vi "Golden Section 1D.vi"(4 "accuracy":dbl=1e-08 format="%.0e", 5 "formula":string="0", 6 "c (start)":dbl format="%.2f", 7 "b (start)":dbl format="%.2f", 8 "a (start)":dbl format="%.2f") -> (0 "error":i32, 1 "ticks":u32, 2 "f(minimum)":dbl format="%.2f", 3 "minimum":dbl format="%.2f")   [LabVIEW 2020, in "NI_Gmath.lvlib"]
doc: "Determines a local minimum of a given 1D function with the help of a bracketing of the minimum. The Golden Section Search method is used."
uses:
  <vilib>/gmath/NI_Gmath.lvlib
panel:
  # "Example:\n\n accuracy: 1E-8 \n a (start): 0.0 \n b (start): 0.5\n c (start): 1.0 \n formula: (x-(3/10))^2+1"
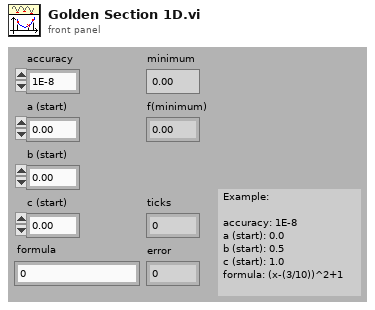
[diagram p1: front panel]
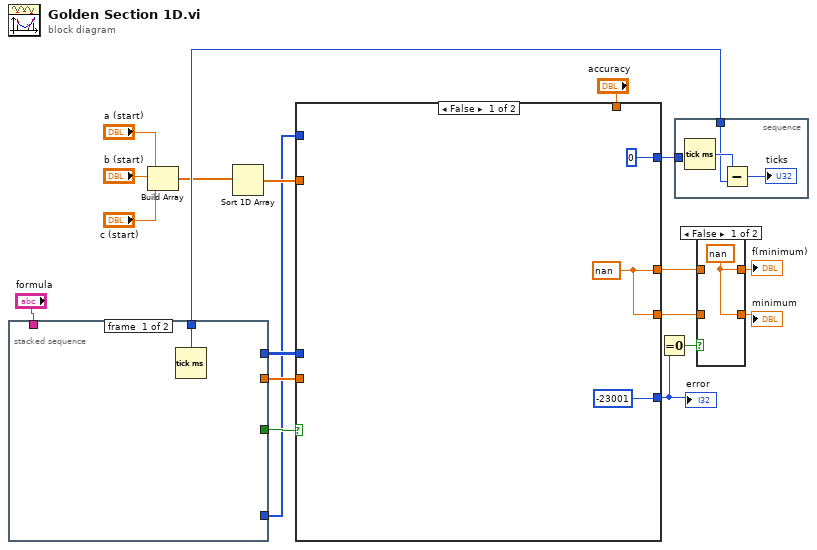
[diagram p0: block diagram]
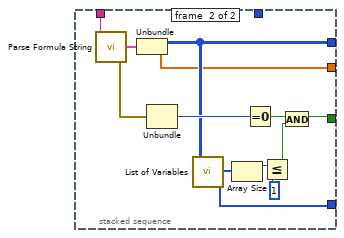
[diagram p3: hidden frame]
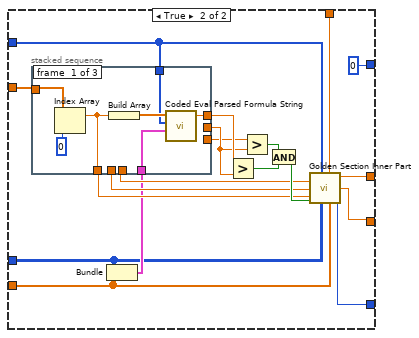
[diagram p4: hidden frame]
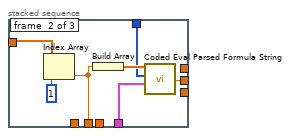
[diagram p5: hidden frame]
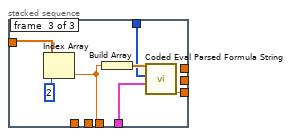
[diagram p6: hidden frame]
diagram:
  n1 = stacked-sequence {
    tunnel: [_ w32] -> w19
    tunnel: [w20 _] -> w18
    tunnel: "formula" -> [_ w26]
    tunnel: [_ w22] -> w3
    tunnel: [_ w21] -> w2
    tunnel: [_ w27] -> w1
    frame #0 {
      n2 = Tick Count (ms)() -> (millisecond timer value=w20:u32)
    }
    frame #1 {
      n3 = call <vilib>:"Parse Formula String.vi"("formula"=w26) -> ("error out"=w25:errorcluster, "Parsed Formula"=w23:cluster{"Table":i32[][], "Y Values":dbl[]})  [unwired: 1 in]
      n4 = Unbundle(w23) -> ("Table"=w22:i32[][], "Y Values"=w21:dbl[])
      n5 = Unbundle(w25) -> ("code"=w24:i32)  [unwired: 2 out]
      n6 = call <vilib>:"List of Variables.vi"("Table"=w22) -> ("List of variables"=w27:i32[])
      n7 = Array Size(array=w27) -> (size(s)=w28:i32)
      n8 = Equal To 0?(x=w24) -> (x = 0?=w31:bool)
      n9 = Less Or Equal?(x=w28, y=1) -> (x <= y?=w30:bool)
      n10 = And(x=w31, y=w30) -> (x .and. y?=w32:bool)
    }
  }
  n11 = Build Array("a (start)", "b (start)", "c (start)") -> (w14:dbl[])
  n12 = Sort 1D Array(array=w14) -> (sorted array=w13:dbl[])
  n13 = case shown="False" w19 {
    tunnel: w13 -> [_ w54]
    tunnel: [0 0] -> w12
    tunnel: [w34 w43] -> w8
    tunnel: [w34 w42] -> w6
    tunnel: [-23001 w41] -> w10
    tunnel: "accuracy" -> [_ w39]
    tunnel: w3 -> [_ w38]
    tunnel: w2 -> [_ w37]
    tunnel: w1 -> [_ w36]
    frame False {
      w34 = nan
      (unwired) 0
    }
    frame True {
      (unwired) 0
      n14 = Bundle("Table"=w38, "Y Values"=w37) -> (w40:cluster{"Table":i32[][], "Y Values":dbl[]})  [unwired: 1 in]
      n15 = stacked-sequence {
        tunnel: w54 -> [w61 w68 w75]
        tunnel: w36 -> [w56 w62 w70]
        tunnel: [w59 _ _] -> w53
        tunnel: [_ w66 _] -> w52
        tunnel: [_ _ w73] -> w51
        tunnel: [w58 _ _] -> w47
        tunnel: [_ w65 _] -> w46
        tunnel: [_ _ w72] -> w45
        tunnel: w40 -> [w55 w63 w69]
        frame #0 {
          n16 = Index Array(array=w61, index=0) -> (element=w58:dbl)
          n17 = Build Array(w58) -> (w57:dbl[])
          n18 = call <vilib>:"Coded Eval Parsed Formula String.vi"("Parsed Formula"=w55, "Variables"=w56, "X Values"=w57) -> ("y value"=w59:dbl)  [unwired: 1 in, 1 out]
        }
        frame #1 {
          n19 = Index Array(array=w68, index=1) -> (element=w65:dbl)
          n20 = Build Array(w65) -> (w64:dbl[])
          n21 = call <vilib>:"Coded Eval Parsed Formula String.vi"("Parsed Formula"=w63, "Variables"=w62, "X Values"=w64) -> ("y value"=w66:dbl)  [unwired: 1 in, 1 out]
        }
        frame #2 {
          n22 = Index Array(array=w75, index=2) -> (element=w72:dbl)
          n23 = Build Array(w72) -> (w71:dbl[])
          n24 = call <vilib>:"Coded Eval Parsed Formula String.vi"("Parsed Formula"=w69, "Variables"=w70, "X Values"=w71) -> ("y value"=w73:dbl)  [unwired: 1 in, 1 out]
        }
      }
      n25 = Greater?(x=w53, y=w52) -> (0:w50:bool)
      n26 = Greater?(x=w51, y=w52) -> (0:w49:bool)
      n27 = And(x=w50, y=w49) -> (x .and. y?=w48:bool)
      n28 = call <vilib>:"Golden Section Inner Part.vi"("result"=w37, "accuracy"=w39, "table"=w38, "case"=w48, "c (start)"=w47, "list of variables"=w36, "b (start)"=w46, "a (start)"=w45) -> ("error"=w41:i32, "f(minimum)"=w42:dbl, "minimum"=w43:dbl)
    }
  }
  "error" <- w10
  n29 = Equal To 0?(x=w10) -> (x = 0?=w9:bool)
  n30 = stacked-sequence {
    tunnel: w18 -> [w77]
    tunnel: w12 -> [_]
    frame #0 {
      n31 = Tick Count (ms)() -> (millisecond timer value=w78:u32)
      n32 = Subtract(x=w78, y=w77) -> (x-y=→"ticks":u32)
    }
  }
  n33 = case shown="False" w9 {
    tunnel: w8 -> [_ w81]
    tunnel: [w79 w81] -> w7
    tunnel: w6 -> [_ w80]
    tunnel: [w79 w80] -> w5
    frame False {
      w79 = nan
    }
    frame True {
    }
  }
  "f(minimum)" <- w7
  "minimum" <- w5
